vi "Append Strings to Log Control.vi"(8 "エラー入力 (エラーなし)":errorcluster, 10 "Appending Strings":string, 11 "Reference to Log Control":refnum<vi>) -> (0 "エラー出力":errorcluster)   [LabVIEW 2014]
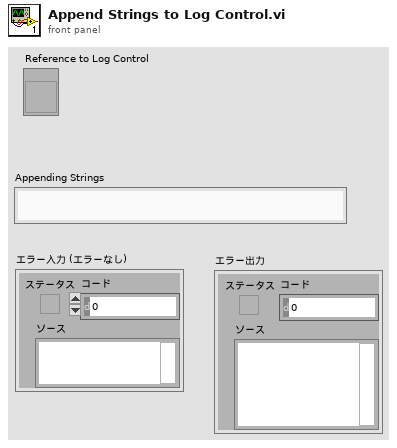
[diagram p1: front panel]
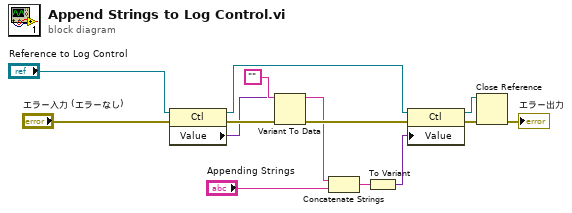
[diagram p0: block diagram]
diagram:
  n1 = property class="Ctl"(reference="Reference to Log Control", error in="エラー入力 (エラーなし)") -> (reference out=w5:refnum<vi>, error out=w12:errorcluster, "Value"=w7:variant)
  n2 = Variant To Data(error in=w12, type="", Variant=w7) -> (data=w8:string, error out=w13:errorcluster)
  n3 = Concatenate Strings(w8, "Appending Strings") -> (w6:string)
  n4 = To Variant(anything=w6) -> (Variant=w14:variant)
  n5 = property class="Ctl"(reference=w5, error in=w13, "Value"=w14) -> (reference out=w10:refnum<vi>, error out=w11:errorcluster)
  n6 = Close Reference(reference=w10, error in (no error)=w11) -> (error out=→"エラー出力":errorcluster)
